vi "subop_x2_Equalization.vi"(0 "Addresses Cluster":T1={"ENA1"=FALSE, "IP address 1"="172.16.14.22", "ENA2"=FALSE, "IP address 2"="172.16.14.23"}, 2 "Equalization parameters":u32[](array[numeric])=[240000, 5, 1600, 900, 100, 4400000, 400000, 2, 0, 99, 2, 40000, 38, 0], 3 "Equalization timeout":u32=2250000000 format="%x", 4 "Global Reg (hex)":u32[](array[numeric])=[68228136, 235670073, 4294967264, 4294967295, 4294967295, 511] format="%x", 5 "PixelReg (hex)":u32[](array[numeric])=[671965161, 384, 671965161, 384, 671965161, 384, 671965161, 384, 671965161, 384, 671965161, 384, 671965161, 384, 671965161, 384, 671965161, 384, 671965161, 384, 671965161, 384, 671965161, 384, 671965161, 384, 671965161, 384, 671965161, 384, 671965161, 384, 671965161, 384, 671965161, 384, 671965161, 384, 671965161, 384, 671965161, 384, 671965161, 384, 671965161, 384, 671965161, 384, 671965161, 384, 671965161, 384, 671965161, 384, 671965161, 384, 671965161, 384, 671965161, 384, 671965161, 384, 671965161, 384, 671965161, 384, 671965161, 384, 671965161, 384, 671965161, 384, 671965161, 384, 671965161, 384, 671965161, 384, 671965161, 384, 671965161, 384, 671965161, 384, 671965161, 384, 671965161, 384, 671965161, 384, 671965161, 384, 671965161, 384, 671965161, 384, 671965161, 384, 671965161, 384, 671965161, 384, 671965161, 384, 671965161, 384, 671965161, 384, 671965161, 384, 671965161, 384, 671965161, 384, 671965161, 384, 671965161, 384, 671965161, 384, 671965161, 384, 671965161, 384, 671965161, 384, 671965161, 384, 671965161, 384, 671965161, 384, 671965161, 384, 671965161, 384, 671965161, 384, 671965161, 384, 671965161, 384, 671965161, 384, 671965161, 384, 671965161, 384, 671965161, 384, 671965161, 384, 671965161, 384, 671965161, 384, 671965161, 384, 671965161, 384, 671965161, 384, 671965161, 384, 671965161, 384, 671965161, 384, 671965161, 384, 671965161, 384, 671965161, 384, 671965161, 384, 671965161, 384, 671965161, 384, 671965161, 384, 671965161, 384, 671965161, 384, 671965161, 384, 671965161, 384, 671965161, 384, 671965161, 384, 671965161, 384, 671965161, 384, 671965161, 384] format="%x") -> (14 "EQ Data and Report":u32[](array[numeric]) format="%x", 16 "timeout or error":bool, 17 "answers done":string, 18 "error out":errorcluster, 19 "EQ timeout":bool)   [LabVIEW 2015, in "VIPM2.lvlib"]
doc: "Equalització: 2xFPGA simultanis amb reentrança.\nEs concatenen els EQ Data and Report."
uses:
  VIPM2.lvlib
panel:
  # "Equalization: 2xFPGA simultaneously"
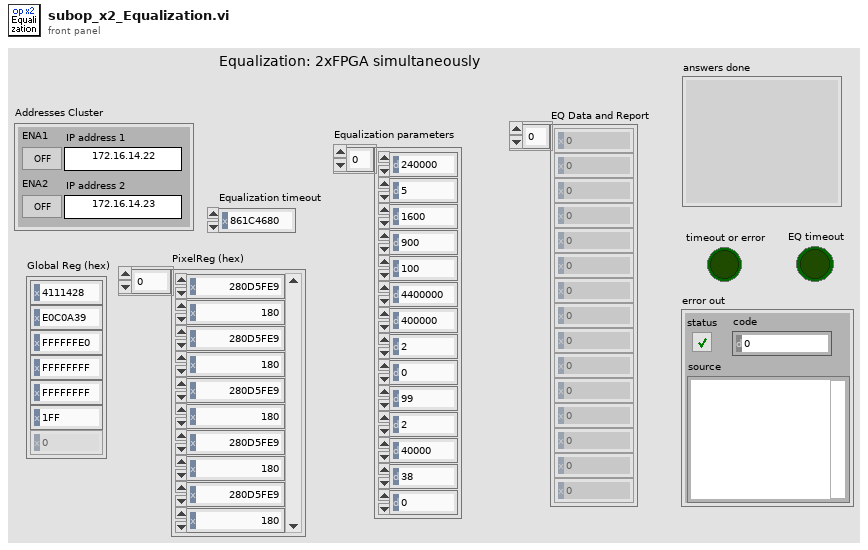
[diagram p1: front panel]
types:
  T1 = cluster{"ENA1":bool, "IP address 1":string, "ENA2":bool, "IP address 2":string}
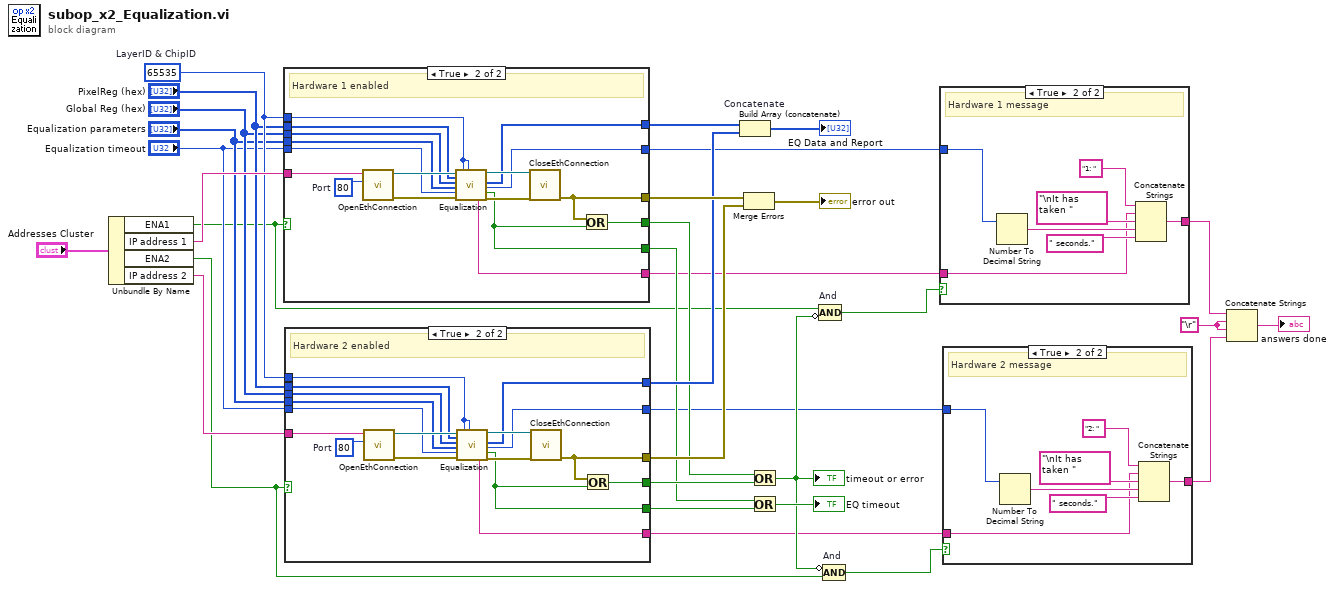
[diagram p0: block diagram]
diagram:
  w3 = "\r"
  w29 = u32 65535  # LayerID & ChipID
  n1 = Unbundle By Name("Addresses Cluster") -> ("ENA1"=w11:bool, "IP address 1"=w31:string, "ENA2"=w8:bool, "IP address 2"=w30:string)
  n2 = case shown="True" w11 {
    tunnel: [_ w45] -> w23
    tunnel: "Equalization timeout" -> [_ w43]
    tunnel: "Equalization parameters" -> [_ w42]
    tunnel: "Global Reg (hex)" -> [_ w41]
    tunnel: "PixelReg (hex)" -> [_ w40]
    tunnel: w29 -> [_ w39]
    tunnel: w31 -> [_ w38]
    tunnel: [_ w37] -> w17
    tunnel: [_ w36] -> w15
    tunnel: [_ w35] -> w12
    tunnel: [_ w34] -> w21
    tunnel: [_ w33] -> w13
    frame False {
      # "Hardware 1 not enabled"
    }
    frame True {
      w44 = u16 80  # Port
      # "Hardware 1 enabled"
      n3 = call "OpenEthConnection.vi"("Port"=w44, "IP address"=w38) -> ("error out"=w48:errorcluster, "connection ID out"=w49:refnum<k5>)  [unwired: 7 in, 1 out]
      n4 = call "Equalization.vi"("connection ID"=w49, "Pixel Register"=w40, "Global Register"=w41, "Equalization parameters"=w42, "Equalization timeout"=w43, "error in (no error)"=w48, "ChipID"=w39, "LayerID"=w39) -> ("Answer"=w35:string, "connection ID out"=w47:refnum<k5>, "EQ Data and Report"=w34:u32[], "EQ time (s)"=w33:u32, "EQ Timeout"=w36:bool, "error out"=w46:errorcluster)  [unwired: 6 in]
      n5 = call "CloseEthConnection.vi"("error in (no error)"=w46, "connection ID"=w47) -> ("error out"=w45:errorcluster)  [unwired: 9 in]
      n6 = Or(x=w45, y=w36) -> (x .or. y?=w37:bool)
    }
  }
  n7 = case shown="True" w8 {
    tunnel: [_ w62] -> w22
    tunnel: "Equalization timeout" -> [_ w60]
    tunnel: "Equalization parameters" -> [_ w59]
    tunnel: "Global Reg (hex)" -> [_ w58]
    tunnel: "PixelReg (hex)" -> [_ w57]
    tunnel: w29 -> [_ w56]
    tunnel: w30 -> [_ w55]
    tunnel: [_ w54] -> w18
    tunnel: [_ w53] -> w16
    tunnel: [_ w52] -> w6
    tunnel: [_ w51] -> w20
    tunnel: [_ w50] -> w5
    frame False {
      # "Hardware 2 not enabled"
    }
    frame True {
      w61 = u16 80  # Port
      # "Hardware 2 enabled"
      n8 = call "OpenEthConnection.vi"("Port"=w61, "IP address"=w55) -> ("error out"=w65:errorcluster, "connection ID out"=w66:refnum<k5>)  [unwired: 7 in, 1 out]
      n9 = call "Equalization.vi"("connection ID"=w66, "Pixel Register"=w57, "Global Register"=w58, "Equalization parameters"=w59, "Equalization timeout"=w60, "error in (no error)"=w65, "ChipID"=w56, "LayerID"=w56) -> ("Answer"=w52:string, "connection ID out"=w64:refnum<k5>, "EQ Data and Report"=w51:u32[], "EQ time (s)"=w50:u32, "EQ Timeout"=w53:bool, "error out"=w63:errorcluster)  [unwired: 6 in]
      n10 = call "CloseEthConnection.vi"("error in (no error)"=w63, "connection ID"=w64) -> ("error out"=w62:errorcluster)  [unwired: 9 in]
      n11 = Or(x=w62, y=w53) -> (x .or. y?=w54:bool)
    }
  }
  n12 = Build Array (concatenate) "Concatenate"(w21, w20) -> (→"EQ Data and Report":u32[])
  n13 = Merge Errors "Merge Errors"(w23, w22) -> (→"error out":errorcluster)
  n14 = Or(x=w17, y=w18) -> (x .or. y?=w9:bool)
  "timeout or error" <- w9
  n15 = Or(x=w15, y=w16) -> (x .or. y?=→"EQ timeout":bool)
  n16 = Compound Arithmetic op=AND "And"(w11, invert w9) -> (w10:bool)
  n17 = Compound Arithmetic op=AND "And"(invert w9, w8) -> (w7:bool)
  n18 = case shown="True" w10 {
    tunnel: w13 -> [_ w70]
    tunnel: w12 -> [_ w68]
    tunnel: [_ w69] -> w4
    frame False {
      # "Hardware 1 not enabled /or/ timeout or error"
    }
    frame True {
      # "Hardware 1 message"
      n19 = Number To Decimal String(number=w70) -> (decimal integer string=w73:string)  [unwired: 1 in]
      n20 = Concatenate Strings("1: " ("string"), w68, "\nIt has taken ", w73, " seconds." ("string")) -> (w69:string)
    }
  }
  n21 = case shown="True" w7 {
    tunnel: w5 -> [_ w77]
    tunnel: w6 -> [_ w75]
    tunnel: [_ w76] -> w2
    frame False {
      # "Hardware 2 not enabled /or/ timeout or error"
    }
    frame True {
      # "Hardware 2 message"
      n22 = Number To Decimal String(number=w77) -> (decimal integer string=w80:string)  [unwired: 1 in]
      n23 = Concatenate Strings("2: " ("string"), w75, "\nIt has taken ", w80, " seconds." ("string")) -> (w76:string)
    }
  }
  n24 = Concatenate Strings "Concatenate Strings"(w4, w3, w3, w2) -> (→"answers done":string)
